vi "ShiftSMPS.vi"(6 "SMPS Sizes":dbl[](array[numeric]), 7 "DeltaX":dbl, 9 "xi used in":dbl[](array[numeric]), 10 "yi in":dbl[](array[numeric]), 11 "Shift in Log scale":dbl) -> (2 "xi used out":dbl[](array[numeric]), 3 "yi out":dbl[](array[numeric]))   [LabVIEW 2013]
doc: "Shift SMPS by the ammount needed so that it aligns with smps selected sizes"
uses:
  <vilib>/gmath/NI_Gmath.lvlib
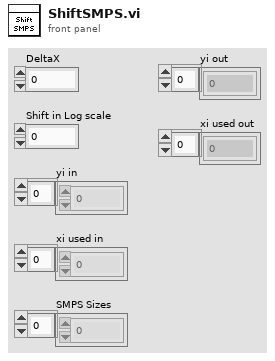
[diagram p1: front panel]
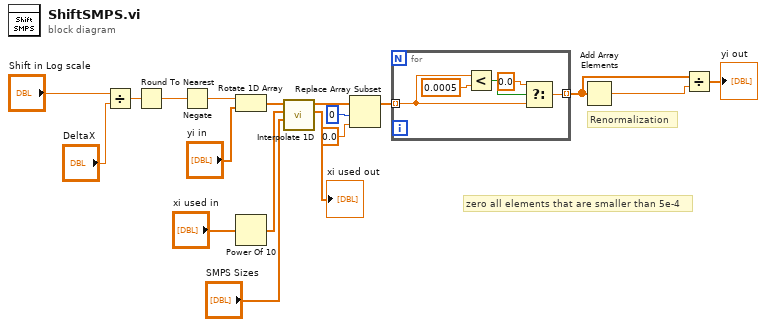
[diagram p0: block diagram]
diagram:
  # "zero all elements that are smaller than 5e-4"
  # "Renormalization"
  n1 = Divide(x="Shift in Log scale", y="DeltaX") -> (x/y=w12:dbl)
  n2 = Round To Nearest(number=w12) -> (nearest integer value=w9:dbl)
  n3 = Negate(x=w9) -> (-x=w8:dbl)
  n4 = Rotate 1D Array(1:"yi in", 2:w8) -> (0:w15:dbl[])
  n5 = Power Of 10(x="xi used in") -> (10^x=w16:dbl[])
  n6 = call <vilib>:"Interpolate 1D.vi"("xi"="SMPS Sizes", "X"=w16, "Y"=w15) -> ("xi used"=→"xi used out":dbl[], "yi"=w7:dbl[])  [unwired: 6 in, 1 out]
  n7 = Replace Array Subset(array=w7, new element=0.0 ("new element/subarray"), index=0) -> (w2:dbl[])
  n8 = for {
    tunnel: w2 -> [w21] mode=indexing
    tunnel: [w19] -> w1 mode=indexing
    n9 = Less?(x=w21, y=0.0005) -> (x < y?=w22:bool)
    n10 = Select(t=0.0, s=w22, f=w21) -> (s? t:f=w19:dbl)
  }
  n11 = Add Array Elements(numeric array=w1) -> (sum=w4:dbl)
  n12 = Divide(x=w1, y=w4) -> (x/y=→"yi out":dbl[])
